vi "MotorSpeedv4.vi"(9 "FirstTime?":bool, 10 "MinPwr":dbl, 11 "MaxPwr":dbl) -> (0 "RightSpdOut":dbl, 2 "Acceled?":bool, 3 "LeftSpdOut":dbl)   [LabVIEW 2017]
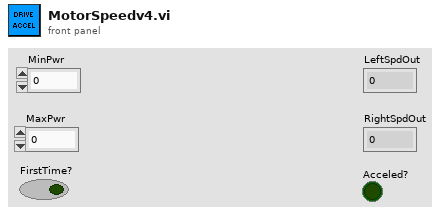
[diagram p1: front panel]
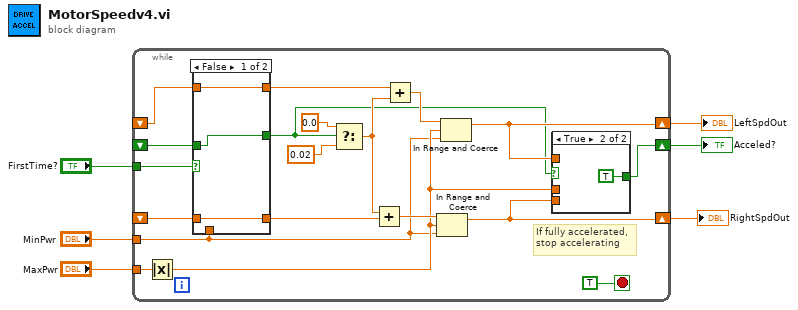
[diagram p0: block diagram]
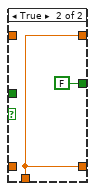
[diagram p2: hidden frame]
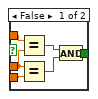
[diagram p3: hidden frame]
diagram:
  n1 = while {
    shift-right: [w25] -> w1
    shift-left: _ -> [w13]
    tunnel: "MaxPwr" -> [w23]
    tunnel: "FirstTime?" -> [w14]
    shift-right: [w20] -> w6
    shift-left: _ -> [w11]
    shift-right: [w17] -> w5
    shift-left: _ -> [w9]
    tunnel: "MinPwr" -> [w7]
    stop <- TRUE stop-if-true
    # "If fully accelerated,\nstop accelerating"
    n2 = Absolute Value(x=w23) -> (abs(x)=w15:dbl)
    n3 = case shown="False" w14 {
      tunnel: w13 -> [w28 _]
      tunnel: [w28 FALSE] -> w12
      tunnel: w11 -> [w27 _]
      tunnel: [w27 w29] -> w10
      tunnel: w9 -> [w26 _]
      tunnel: [w26 w29] -> w8
      tunnel: w7 -> [_ w29]
      frame False {
      }
      frame True {
      }
    }
    n4 = Select(t=0.0, s=w12, f=0.02 ("t")) -> (s? t:f=w19:dbl)
    n5 = Add(x=w19, y=w8) -> (x+y=w16:dbl)
    n6 = Add(x=w10, y=w19) -> (x+y=w18:dbl)
    n7 = In Range and Coerce(upper limit=w16, x=w15, lower limit=w7) -> (coerced(x)=w17:dbl)  [unwired: 1 out]
    n8 = In Range and Coerce(upper limit=w18, x=w15, lower limit=w7) -> (coerced(x)=w20:dbl)  [unwired: 1 out]
    n9 = case shown="True" w12 {
      tunnel: w20 -> [w36 _]
      tunnel: w17 -> [w35 _]
      tunnel: [w34 TRUE] -> w25
      tunnel: w15 -> [w33 _]
      frame False {
        n10 = Equal?(x=w36, y=w33) -> (x = y?=w32:bool)
        n11 = Equal?(x=w33, y=w35) -> (x = y?=w31:bool)
        n12 = And(x=w32, y=w31) -> (x .and. y?=w34:bool)
      }
      frame True {
      }
    }
  }
  "LeftSpdOut" <- w6
  "RightSpdOut" <- w5
  "Acceled?" <- w1
